vi "Launch Aggregate Model (Explicit).vi"(8 "error in (no error)":errorcluster, 10 "Model to Launch":refnum<class "IModel.lvclass">, 11 "IModel in":refnum<class "IModel.lvclass">) -> (0 "error out":errorcluster, 2 "Nested Model's Enqueuer":refnum<class "Message Enqueuer.lvclass">, 3 "IModel out":refnum<class "IModel.lvclass">)   [LabVIEW 2015, in "IModel.lvlib" / "IModel.lvclass"]
uses:
  IModel.lvclass
  <vilib>/ActorFramework/Message Enqueuer/Message Enqueuer.lvclass
  IModel.lvclass/IModel.ctl
  <vilib>/ActorFramework/Actor/Actor.lvclass
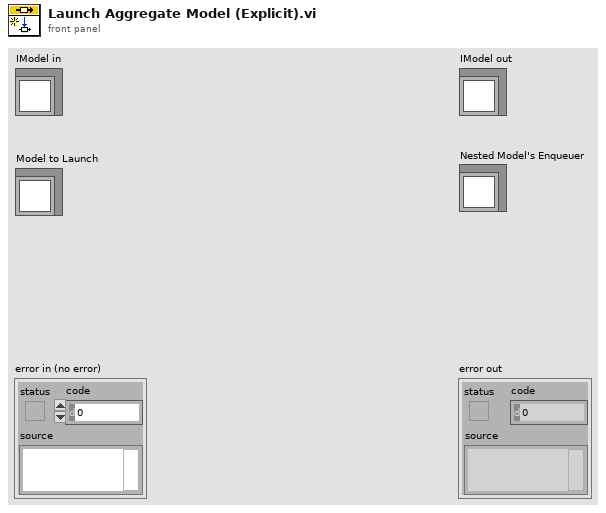
[diagram p1: front panel]
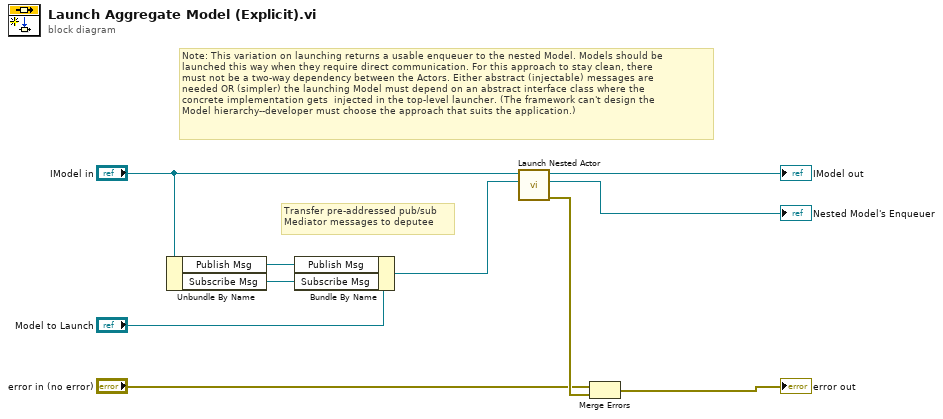
[diagram p0: block diagram]
diagram:
  # "Transfer pre-addressed pub/sub\nMediator messages to deputee"
  # "Note: This variation on launching returns a usable enqueuer to the nested Model. Models should be\nlaunched this way when they require direct communication. For this approach to stay clean, there\nmust not be a two-way dependency between the Actors. Either abstract (injectable) messages are\nneeded OR (simpler) the launching Model must depend on an abstract interface class where the\nconcrete implementation gets  injected in the top-level launcher. (The framework can't design the\nModel hierarchy--developer must choose the approach that suits the application.)"
  n1 = Unbundle By Name("IModel in") -> ("Publish Msg"=w4:refnum<class "Publish Msg.lvclass">, "Subscribe Msg"=w3:refnum<class "Subscribe Msg.lvclass">)
  n2 = Bundle By Name(cluster="Model to Launch", "Publish Msg"=w4, "Subscribe Msg"=w3) -> (w2:refnum<class "IModel.lvclass">)
  n3 = call <vilib>:"Launch Nested Actor.vi"("Nested Actor"=w2, "Caller Actor in"="IModel in") -> ("error out"=w8:errorcluster, "Nested Actor's Enqueuer"=→"Nested Model's Enqueuer":refnum<class "Message Enqueuer.lvclass">, "Caller Actor out"=→"IModel out":refnum<class "IModel.lvclass">)  [unwired: 7 in]
  n4 = Merge Errors("error in (no error)", w8) -> (→"error out":errorcluster)
